vi "data_savetxt_demo.vi"() -> ()   [LabVIEW 2022 SP3]
panel:
  in  "stop":bool
  out "path_out":path
  in  "Save":bool
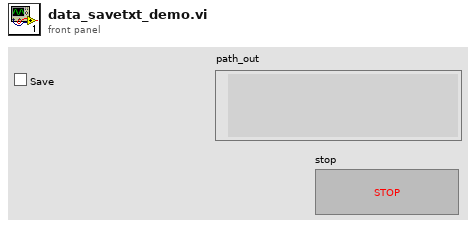
[diagram p1: front panel]
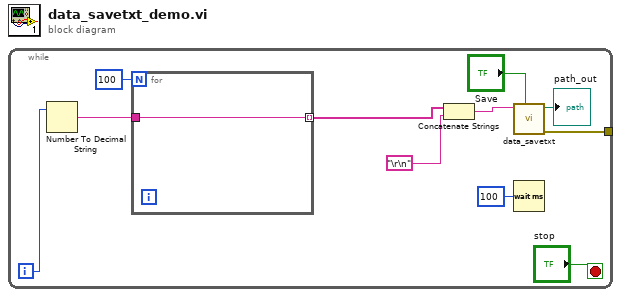
[diagram p0: block diagram]
diagram:
  n1 = while {
    tunnel: [w6] -> _
    i -> [w11]
    stop <- "stop" stop-if-true
    n2 = Number To Decimal String(number=w11) -> (decimal integer string=w3:string)  [unwired: 1 in]
    n3 = for {
      N: 100 -> [_]
      tunnel: [w12] -> w2 mode=indexing
      tunnel: w3 -> [w12]
    }
    n4 = Concatenate Strings(w2, "\r\n") -> (w5:string)
    n5 = call "data_savetxt.vi"("Save"="Save", "ParasOutput"=w5) -> ("error out"=w6:errorcluster, "path_out"=→"path_out":path)  [unwired: 8 in]
    n6 = Wait (ms)(milliseconds to wait=u32 100) -> ()  [unwired: 1 out]
  }
